vi "Initialize DMM.vi"(6 "initialize and close session behavior":T1, 8 "error in (no error)":errorcluster, 10 "reset":bool, 11 "KeysightDmm in":refnum<class "KeysightDmm.lvclass">) -> (0 "error out":errorcluster, 3 "KeysightDmm out":refnum<class "KeysightDmm.lvclass">)   [LabVIEW 2021, in "KeysightDmm.lvclass"]
doc: "Initializes the driver session for KeysightDmm."
uses:
  KeysightDmm.lvclass
  C:/Program Files/National Instruments/LabVIEW 2021/vi.lib/Plug-In SDKs/Sessions/Instrument/ISession Factory/ISession Factory.lvclass
  <vilib>/Plug-In SDKs/Clients/Session Management V1/Session Reservation/Initialize and Close Session Behavior.ctl
  KeysightDmm.lvclass/KeysightDmm.ctl
  8196af0f-1c90-4534-837c-d451b2e8b892.vi
  <vilib>/Plug-In SDKs/Clients/Session Management V1/Session Reservation/Initialize Sessions with Retry.vi
  <vilib>/Plug-In SDKs/Clients/Session Management V1/Session Reservation/Session Reservation.lvclass
panel:
  out "channel list":string
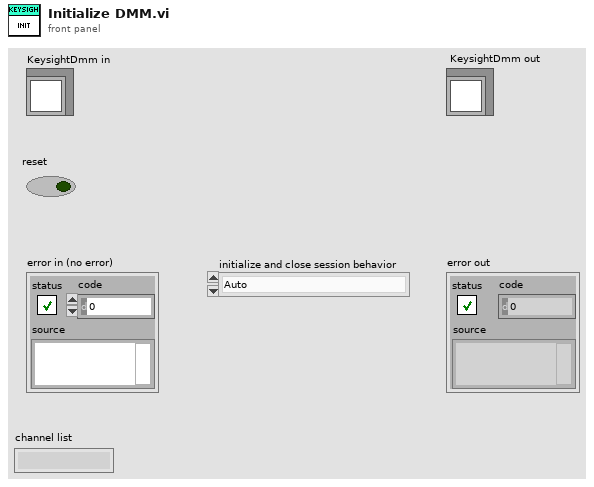
[diagram p1: front panel]
types:
  T1 = typedef "NI Session Management V1 Client.lvlib/Session Reservation.lvclass/Initialize and Close Session Behavior.ctl" = enum16{"Auto", "Initialize and Close", "Attach and Detach", "Initialize and Detach", "Attach and Close"}
  T2 = cluster{"Baud Rate":u32, "Parity":u16, "Data Bits":u16}
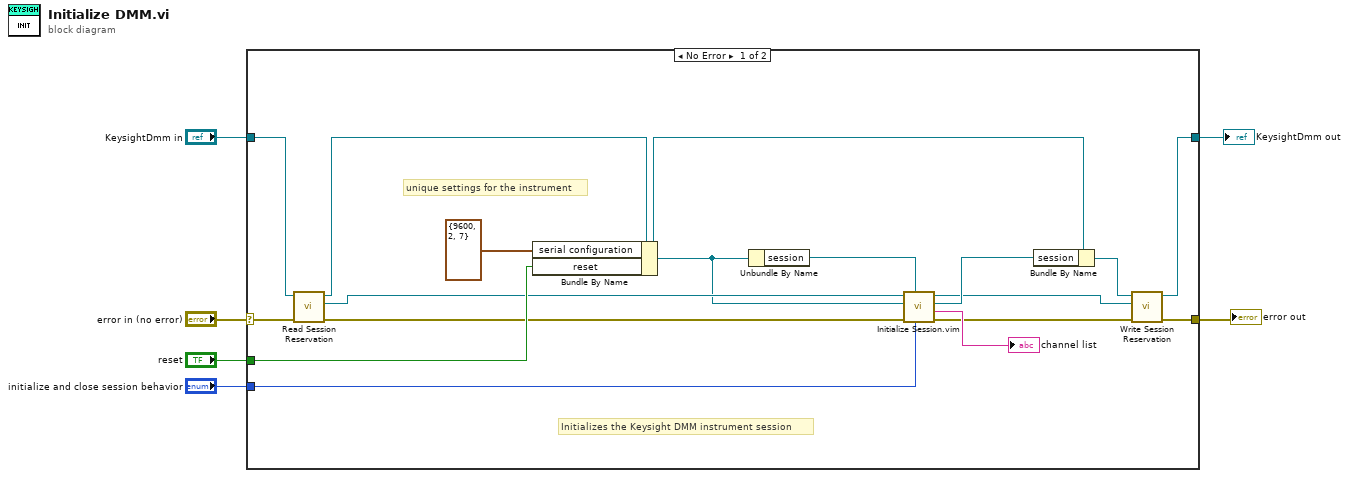
[diagram p0: block diagram]
diagram:
  n1 = case shown="No Error" "error in (no error)" {
    selector: "error in (no error)" -> [w17 w24]
    tunnel: [w13 w24] -> w5
    tunnel: [w11 w25] -> w4
    tunnel: "KeysightDmm in" -> [w8 w25]
    tunnel: "reset" -> [w20 _]
    tunnel: "initialize and close session behavior" -> [w19 _]
    frame No Error {
      # "Initializes the Keysight DMM instrument session"
      # "unique settings for the instrument"
      n2 = call-dynamic "Read Session Reservation.vi"("error in (no error)"=w17, "DMM_Base in"=w8) -> ("error out"=w16:errorcluster, "Session Reservation"=w15:refnum<class "Session Reservation.lvclass">, "DMM_Base out"=w9:refnum<class "KeysightDmm.lvclass">)  [unwired: 7 in]
      n3 = Bundle By Name(cluster=w9, "serial configuration"=T2 {"Baud Rate"=9600, "Parity"=2, "Data Bits"=7}, "reset"=w20) -> (w7:refnum<class "KeysightDmm.lvclass">)
      n4 = Unbundle By Name(w7) -> ("session"=w21:refnum<visa-resource-name>)
      n5 = call "Initialize Session.vim"("initialize and close session behavior"=w19, "session type"=w21, "error in"=w16, "session factory"=w7, "session reservation in"=w15) -> ("error out"=w14:errorcluster, "channel list"=→"channel list":string, "session"=w18:refnum<visa-resource-name>, "session reservation out"=w10:refnum<class "Session Reservation.lvclass">)  [unwired: 3 in]
      n6 = Bundle By Name(cluster=w7, "session"=w18) -> (w12:refnum<class "KeysightDmm.lvclass">)
      n7 = call-dynamic "Write Session Reservation.vi"("error in (no error)"=w14, "Session Reservation"=w10, "DMM_Base in"=w12) -> ("error out"=w13:errorcluster, "DMM_Base out"=w11:refnum<class "KeysightDmm.lvclass">)  [unwired: 7 in]
    }
    frame Error {
    }
  }
  "error out" <- w5
  "KeysightDmm out" <- w4
